vi "TE.vi"(8 "error in (no error)":errorcluster, 10 "Retries":i32, 11 "Agilis in":T1) -> (0 "error out":errorcluster, 3 "Agilis out":T1)   [LabVIEW 2016, in "Drivers.lvlib" / "Agilis.lvlib"]
doc: "Returns the error code of the previous command. Each command generates an error code including \"0\" for NO ERROR. This error code can be queried with the TE command. For a safe program, it is recommended to always query the command error after each command execution."
uses:
  Agilis.lvlib
  AgilisCmdLib Refnum.ctl
  C:/Users/MyUser/Desktop/Trace Grabber/Drivers/Agilis/AgilisCmdLib.dll
  AgilisCmdLib.dll
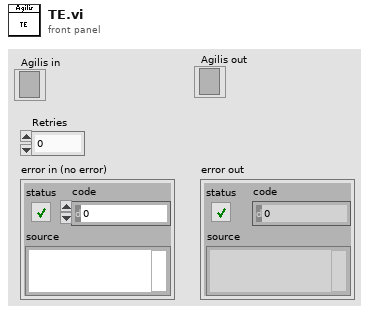
[diagram p1: front panel]
types:
  T1 = typedef "Drivers.lvlib/Agilis.lvlib/AgilisCmdLib Refnum.ctl" = refnum<k24>
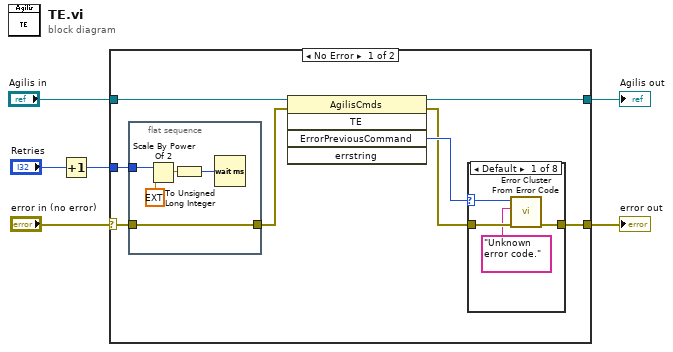
[diagram p0: block diagram]
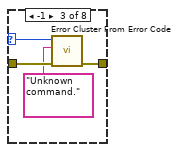
[diagram p3: hidden frame]
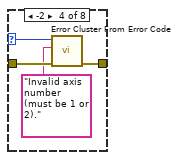
[diagram p4: hidden frame]
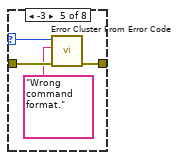
[diagram p5: hidden frame]
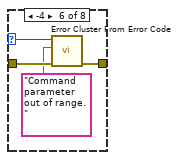
[diagram p6: hidden frame]
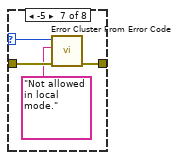
[diagram p7: hidden frame]
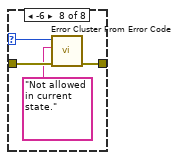
[diagram p8: hidden frame]
diagram:
  n1 = Increment(x="Retries") -> (x+1=w1:i32)
  n2 = case shown="No Error" "error in (no error)" {
    selector: "error in (no error)" -> [w8 w50]
    tunnel: "Agilis in" -> [w14 w49]
    tunnel: [w13 w49] -> w4
    tunnel: [w12 w50] -> w3
    tunnel: w1 -> [w7 _]
    frame No Error {
      n3 = flat-sequence {
        tunnel: [w19] -> w9
        tunnel: w8 -> [w19]
        tunnel: w7 -> [w17]
        frame #0 {
          n4 = Scale By Power Of 2(n=w17, x=ext 10.0) -> (x*2^n=w15:ext)
          n5 = To Unsigned Long Integer(number=w15) -> (unsigned 32bit integer=w18:u32)
          n6 = Wait (ms)(milliseconds to wait=w18) -> ()  [unwired: 1 out]
        }
      }
      n7 = invoke class="AgilisCmds" method="TE"(reference=w14, error in=w9) -> (reference out=w13:T1, error out=w10:errorcluster, "ErrorPreviousCommand"=w11:i32)  [unwired: 3 in, 2 out]
      n8 = case shown="Default" w11 {
        selector: w11 -> [w21 _ w26 w30 w34 w38 w42 w46]
        tunnel: [w23 w24 w28 w32 w36 w40 w44 w48] -> w12
        tunnel: w10 -> [w22 w24 w27 w31 w35 w39 w43 w47]
        frame Default {
          n9 = call <vilib>:"Error Cluster From Error Code.vi"("error in (no error)"=w22, "error message (\"\")"="Unknown error code." ("error message (\"\")"), "error code (0)"=w21) -> ("error out"=w23:errorcluster)  [unwired: 6 in]
        }
        frame 0 {
        }
        frame -1 {
          n10 = call <vilib>:"Error Cluster From Error Code.vi"("error in (no error)"=w27, "error message (\"\")"="Unknown command." ("error message (\"\")"), "error code (0)"=w26) -> ("error out"=w28:errorcluster)  [unwired: 6 in]
        }
        frame -2 {
          n11 = call <vilib>:"Error Cluster From Error Code.vi"("error in (no error)"=w31, "error message (\"\")"="Invalid axis number (must be 1 or 2)." ("error message (\"\")"), "error code (0)"=w30) -> ("error out"=w32:errorcluster)  [unwired: 6 in]
        }
        frame -3 {
          n12 = call <vilib>:"Error Cluster From Error Code.vi"("error in (no error)"=w35, "error message (\"\")"="Wrong command format." ("error message (\"\")"), "error code (0)"=w34) -> ("error out"=w36:errorcluster)  [unwired: 6 in]
        }
        frame -4 {
          n13 = call <vilib>:"Error Cluster From Error Code.vi"("error in (no error)"=w39, "error message (\"\")"="Command parameter out of range." ("error message (\"\")"), "error code (0)"=w38) -> ("error out"=w40:errorcluster)  [unwired: 6 in]
        }
        frame -5 {
          n14 = call <vilib>:"Error Cluster From Error Code.vi"("error in (no error)"=w43, "error message (\"\")"="Not allowed in local mode." ("error message (\"\")"), "error code (0)"=w42) -> ("error out"=w44:errorcluster)  [unwired: 6 in]
        }
        frame -6 {
          n15 = call <vilib>:"Error Cluster From Error Code.vi"("error in (no error)"=w47, "error message (\"\")"="Not allowed in current state." ("error message (\"\")"), "error code (0)"=w46) -> ("error out"=w48:errorcluster)  [unwired: 6 in]
        }
      }
    }
    frame Error {
    }
  }
  "Agilis out" <- w4
  "error out" <- w3
